vi "Inverse DST.vi"   [LabVIEW 2020, in "NI_AALPro.lvlib"]
doc: "Computes the inverse Discrete Sine Transform (DST) of the input sequence <B>DST {X}</B>. Wire data to the <B>DST {X}</B> input to determine the polymorphic instance to use or manually select the instance."
uses:
  <vilib>/Analysis/NI_AALPro.lvlib
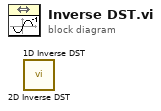
[diagram p0: block diagram]
diagram:
  n1 = call <vilib>:"2D Inverse DST.vi"() -> ()  [unwired: 10 in, 2 out]
  n2 = call <vilib>:"1D Inverse DST.vi"() -> ()  [unwired: 10 in, 2 out]
